vi "MSET.vi"(0 "refnum in":refnum<vi>, 1 "Keys":string[](array[string]), 5 "Values":string[](array[string]), 11 "error in":errorcluster) -> (4 "refnum out":refnum<vi>, 6 "Data":T1, 15 "error out":errorcluster)   [LabVIEW 2020]
uses:
  SubVIs/Controls/redis-data.ctl
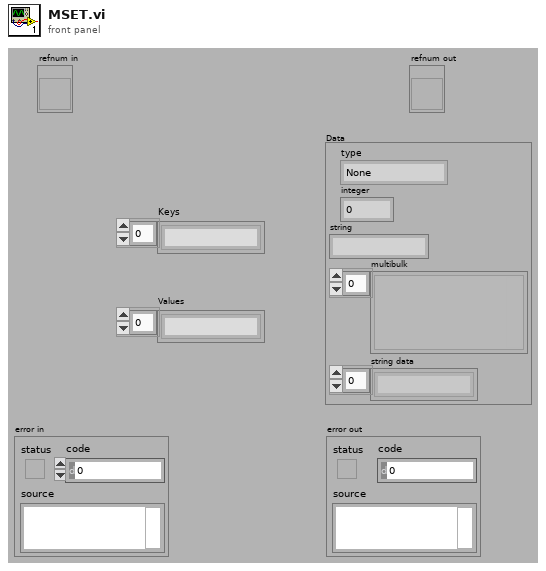
[diagram p1: front panel]
types:
  T1 = typedef "redis-data.ctl" = cluster{"type":enum16{"None", "Error", "Status", "Nil", "Integer", "String", "Multibulk"}, "integer":i64, "string":string, "multibulk":variant[], "string data":string[]}
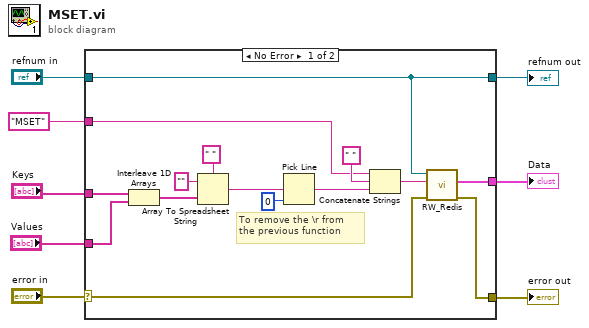
[diagram p0: block diagram]
diagram:
  n1 = case shown="No Error" "error in" {
    selector: "error in" -> [w15 w25]
    tunnel: "Keys" -> [w10 _]
    tunnel: "MSET" -> [w17 _]
    tunnel: "refnum in" -> [w12 w24]
    tunnel: [w14 w25] -> w4
    tunnel: [w13 _] -> w3
    tunnel: [w12 w24] -> w2
    tunnel: "Values" -> [w11 _]
    frame No Error {
      # "To remove the \\r from\nthe previous function"
      n2 = Interleave 1D Arrays(w10, w11) -> (w9:string[])
      n3 = Array To Spreadsheet String(delimiter (Tab)=" ", array=w9, 3:"" ("format string")) -> (spreadsheet string=w19:string)
      n4 = Pick Line(multi-line string=w19, line index=0) -> (output string=w20:string)  [unwired: 1 in]
      n5 = Concatenate Strings(w17, " ", w20) -> (w16:string)
      n6 = call "RW_Redis.vi"("error in"=w15, "command"=w16, "refnum"=w12) -> ("error out"=w14:errorcluster, "Data"=w13:T1)  [unwired: 7 in]
    }
    frame Error {
    }
  }
  "error out" <- w4
  "Data" <- w3
  "refnum out" <- w2
